vi "aplication 2.vi"() -> ()   [LabVIEW 2019]
panel:
  out "Waveform Graph":dbl[](graph)
  out "XY Graph":cluster{dbl[], dbl[]}(graph)
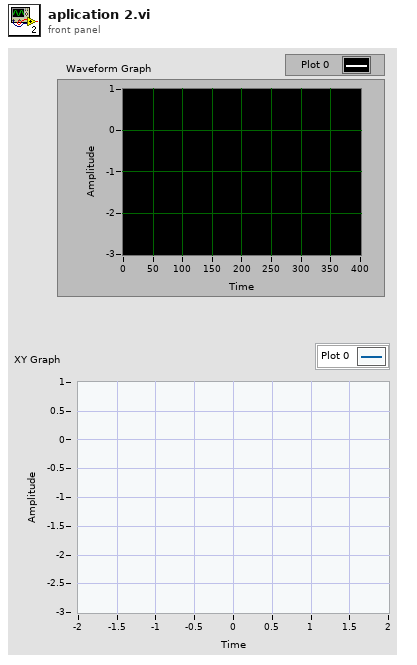
[diagram p1: front panel]
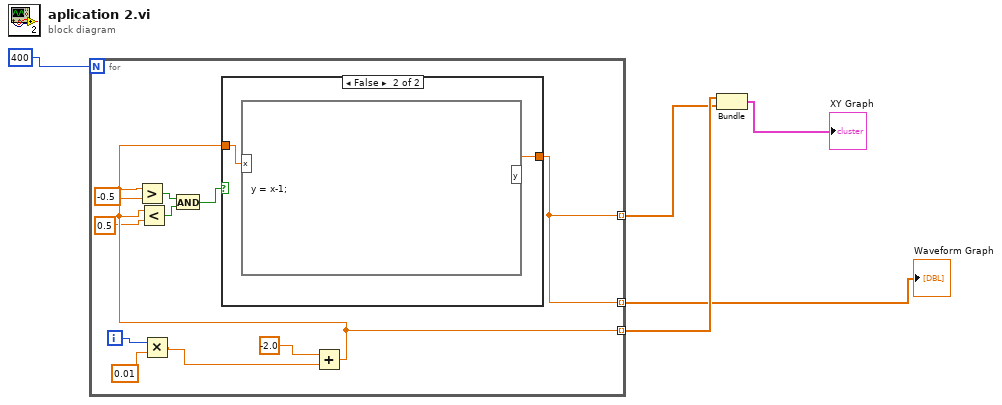
[diagram p0: block diagram]
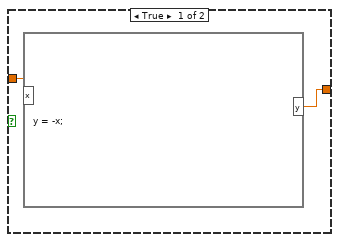
[diagram p2: hidden frame]
diagram:
  n1 = for {
    N: 400 -> [_]
    tunnel: [w8] -> w4 mode=indexing
    tunnel: [w15] -> w3 mode=indexing
    tunnel: [w15] -> w1 mode=indexing
    i -> [w14]
    n2 = Multiply(x=w14, y=0.01) -> (x*y=w12:dbl)
    n3 = Add(x=-2.0, y=w12) -> (x+y=w8:dbl)
    n4 = Greater?(x=w8, y=-0.5) -> (0:w10:bool)
    n5 = Less?(x=w8, y=0.5) -> (x < y?=w9:bool)
    n6 = And(x=w10, y=w9) -> (x .and. y?=w11:bool)
    n7 = case shown="False" w11 {
      tunnel: w8 -> [w18 w20]
      tunnel: [w17 w19] -> w15
      frame True {
        n8 = formula code="y = -x;"("x"=w18) -> ("y"=w17:dbl)
      }
      frame False {
        n9 = formula code="y = x-1;"("x"=w20) -> ("y"=w19:dbl)
      }
    }
  }
  "Waveform Graph" <- w1
  n10 = Bundle(w4, w3) -> (→"XY Graph":cluster{dbl[], dbl[]})  [unwired: 1 in]
